vi "Unscale and Scale - 8 Bit.vi"(8 "error in (no error)":errorcluster, 11 "Data Scaling in":refnum<class "Data Scaling.lvclass">) -> (0 "error out":errorcluster, 3 "Data Scaling out":refnum<class "Data Scaling.lvclass">)   [LabVIEW 2020, in "Unit Tests.lvlib" / "Data Scaling.lvclass"]
uses:
  Data Scaling.lvclass
  Frames & Messages/TypeDefs/Scaling Information.ctl
  Frames & Messages/Utility/Scale Data.vi
  Frames & Messages/Utility/Unscale Data.vi
  <vilib>/addons/_JKI Toolkits/Caraya/classes/Assert/Assert True.vi
  <vilib>/addons/_JKI Toolkits/Caraya/classes/Test/Test.lvclass
  BCI-1553 API.lvlib
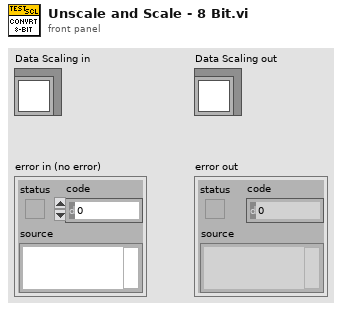
[diagram p1: front panel]
types:
  T1 = typedef "BCI-1553 API.lvlib/Scaling Information.ctl" = cluster{"Bit Offset":i32, "Bit Count":i32, "LSB Resolution":dbl, "2's Complement":bool, "Big Endian":bool, "Sign Bit":bool}
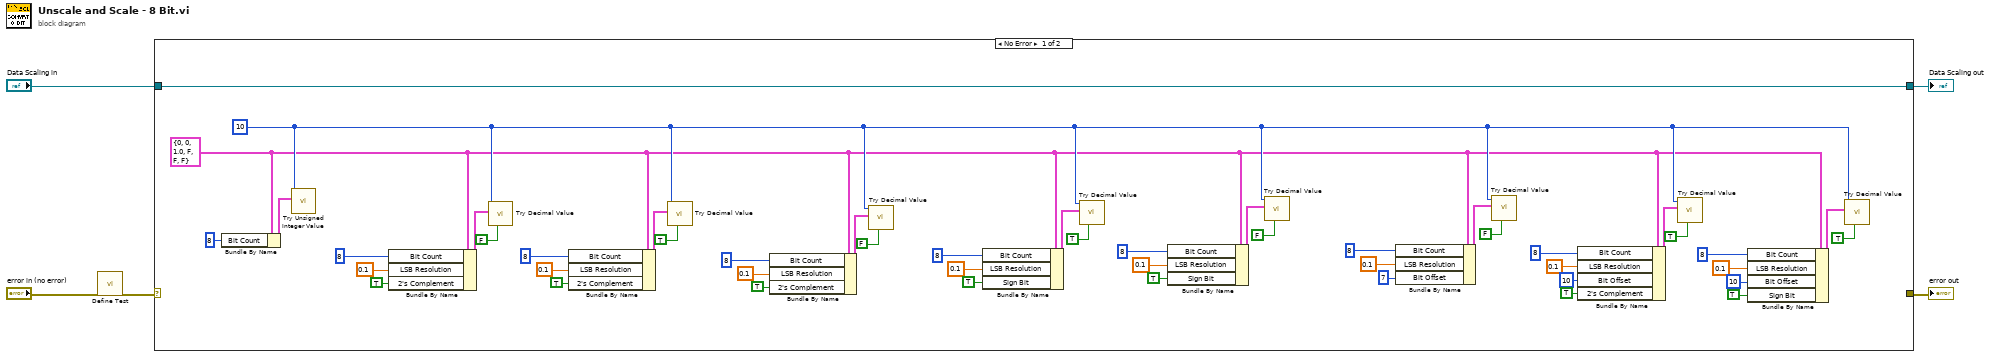
[diagram p0: block diagram]
diagram:
  n1 = call <vilib>:"Define Test.vi"("error in (no error)"="error in (no error)") -> ("error out"=w1:errorcluster)  [unwired: 9 in, 1 out]
  n2 = case shown="No Error" w1 {
    selector: w1 -> [_ w54]
    tunnel: [_ w54] -> w5
    tunnel: [w52 w53] -> w3
    tunnel: "Data Scaling in" -> [w52 w53]
    frame No Error {
      w6 = T1 {"Bit Offset"=0, "Bit Count"=0, "LSB Resolution"=1.0, "2's Complement"=FALSE, "Big Endian"=FALSE, "Sign Bit"=FALSE} ("Scaling Info")
      w7 = 10 ("Random Attempts")
      n3 = Bundle By Name(cluster=w6, "Bit Count"=8) -> (w30:T1)
      n4 = call "Try Unsigned Integer Value.vi"("Scaling Info"=w30, "Random Attempts"=w7) -> ()  [unwired: 9 in, 1 out]
      n5 = Bundle By Name(cluster=w6, "Bit Count"=8, "LSB Resolution"=0.1, "2's Complement"=TRUE) -> (w27:T1)
      n6 = call "Try Decimal Value.vi"("Negate?"=FALSE, "Scaling Info"=w27, "Random Attempts"=w7) -> ()  [unwired: 8 in, 1 out]
      n7 = Bundle By Name(cluster=w6, "Bit Count"=8, "LSB Resolution"=0.1, "2's Complement"=TRUE) -> (w32:T1)
      n8 = call "Try Decimal Value.vi"("Negate?"=TRUE, "Scaling Info"=w32, "Random Attempts"=w7) -> ()  [unwired: 8 in, 1 out]
      n9 = Bundle By Name(cluster=w6, "Bit Count"=8, "LSB Resolution"=0.1, "2's Complement"=TRUE) -> (w37:T1)
      n10 = call "Try Decimal Value.vi"("Negate?"=FALSE, "Scaling Info"=w37, "Random Attempts"=w7) -> ()  [unwired: 8 in, 1 out]
      n11 = Bundle By Name(cluster=w6, "Bit Count"=8, "LSB Resolution"=0.1, "Sign Bit"=TRUE ("2's Complement")) -> (w10:T1)
      n12 = call "Try Decimal Value.vi"("Negate?"=TRUE, "Scaling Info"=w10, "Random Attempts"=w7) -> ()  [unwired: 8 in, 1 out]
      n13 = Bundle By Name(cluster=w6, "Bit Count"=8, "LSB Resolution"=0.1, "Sign Bit"=TRUE ("2's Complement")) -> (w20:T1)
      n14 = call "Try Decimal Value.vi"("Negate?"=FALSE, "Scaling Info"=w20, "Random Attempts"=w7) -> ()  [unwired: 8 in, 1 out]
      n15 = Bundle By Name(cluster=w6, "Bit Count"=8, "LSB Resolution"=0.1, "Bit Offset"=7) -> (w16:T1)
      n16 = call "Try Decimal Value.vi"("Negate?"=FALSE, "Scaling Info"=w16, "Random Attempts"=w7) -> ()  [unwired: 8 in, 1 out]
      n17 = Bundle By Name(cluster=w6, "Bit Count"=8, "LSB Resolution"=0.1, "Bit Offset"=10, "2's Complement"=TRUE) -> (w49:T1)
      n18 = call "Try Decimal Value.vi"("Negate?"=TRUE, "Scaling Info"=w49, "Random Attempts"=w7) -> ()  [unwired: 8 in, 1 out]
      n19 = Bundle By Name(cluster=w6, "Bit Count"=8, "LSB Resolution"=0.1, "Bit Offset"=10, "Sign Bit"=TRUE ("2's Complement")) -> (w42:T1)
      n20 = call "Try Decimal Value.vi"("Negate?"=TRUE, "Scaling Info"=w42, "Random Attempts"=w7) -> ()  [unwired: 8 in, 1 out]
    }
    frame Error {
    }
  }
  "error out" <- w5
  "Data Scaling out" <- w3
